vi "TempAlgoTest (SubVI).vi"(0 "Temp":refnum<vi>, 1 "Speed Ind":dbl format="%#_13g", 2 "Motor Speed RPM":refnum<vi>, 3 "Round":T1(ring), 4 "Temp Up In":dbl format="%#_13g", 5 "error in (no error)":errorcluster, 6 "String in":refnum<vi>, 7 "Temp Goal":dbl format="%#_13g", 8 "Stop":refnum<vi>, 9 "Speed Goal":dbl format="%#_13g", 10 "Stop BurnIn":refnum<vi>, 11 "AD Resistor Step":i32=9, 12 "Strin":string, 13 "AccuTemp":dbl=3.0 format="%#_13g") -> (14 "Speed Pass/Fail":bool, 15 "Temp  Pass/Fail":dbl, 16 "Temp Up Out":dbl, 17 "Speed Pass/Fail":dbl, 18 "Temp Pass/Fail":bool, 19 "error out":errorcluster)   [LabVIEW 2017]
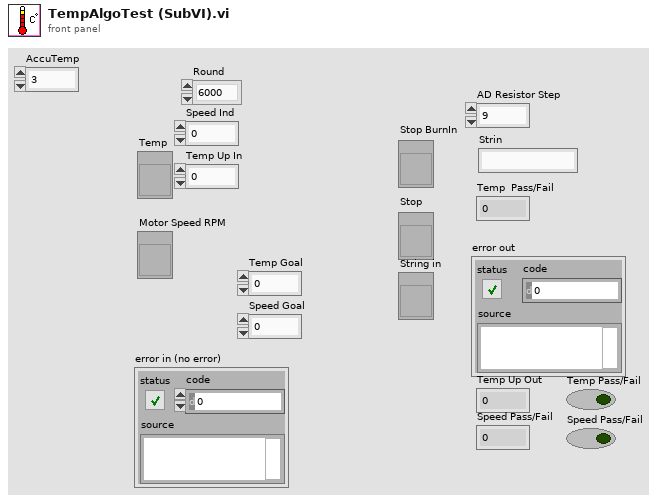
[diagram p1: front panel]
types:
  T1 = enum32{"6000", "11500", "15100", "11500-2", "6000-2"}
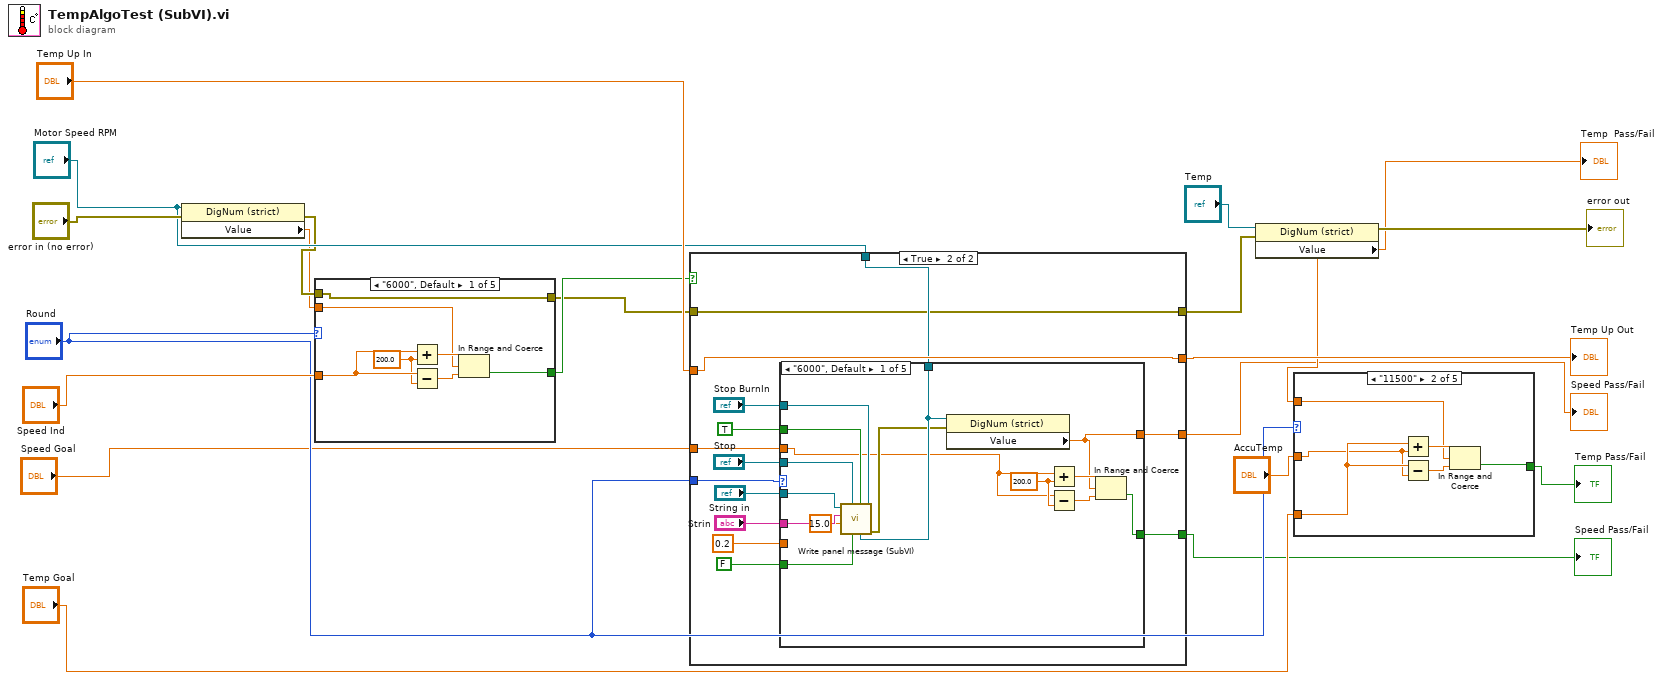
[diagram p0: block diagram]
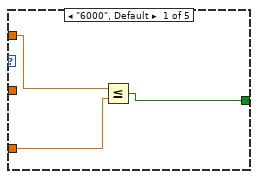
[diagram p2: hidden frame]
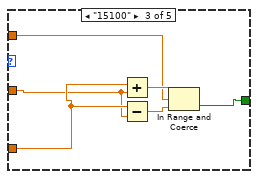
[diagram p3: hidden frame]
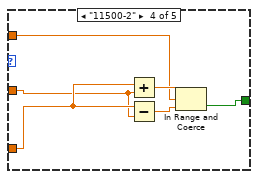
[diagram p4: hidden frame]
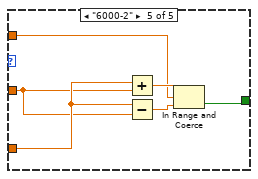
[diagram p5: hidden frame]
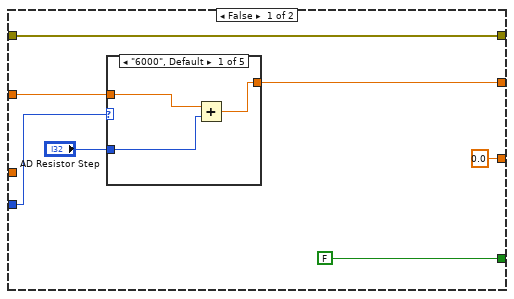
[diagram p6: hidden frame]
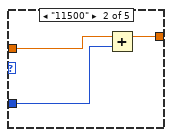
[diagram p7: hidden frame]
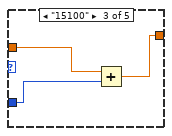
[diagram p8: hidden frame]
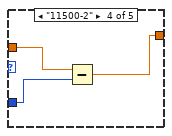
[diagram p9: hidden frame]
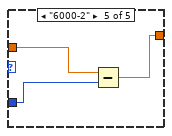
[diagram p10: hidden frame]
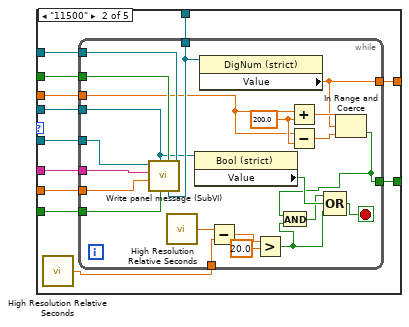
[diagram p11: hidden frame]
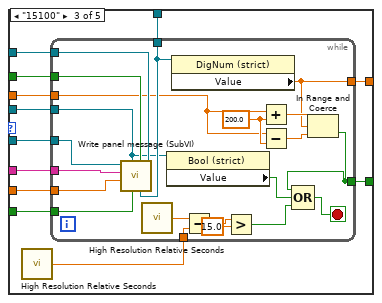
[diagram p12: hidden frame]
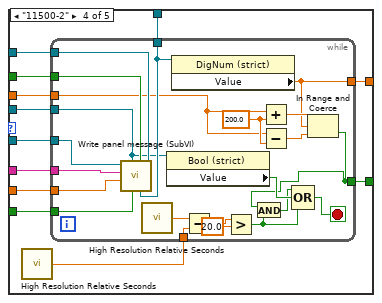
[diagram p13: hidden frame]
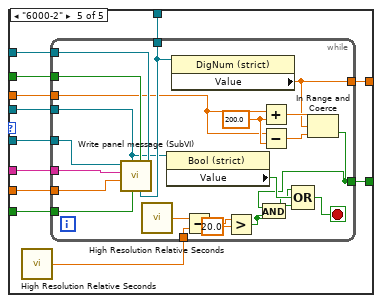
[diagram p14: hidden frame]
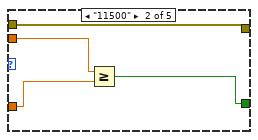
[diagram p15: hidden frame]
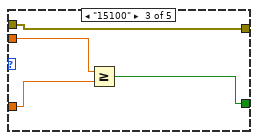
[diagram p16: hidden frame]
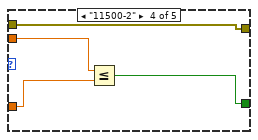
[diagram p17: hidden frame]
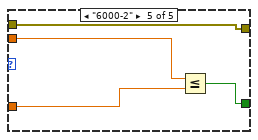
[diagram p18: hidden frame]
diagram:
  n1 = property class="DigNum (strict)"(reference="Motor Speed RPM", error in="error in (no error)") -> (error out=w7:errorcluster, "Value"=w4:dbl)  [unwired: 1 out]
  n2 = case shown="\"6000\", Default" "Round" {
    tunnel: w4 -> [w24 w31 w35 w39 w43]
    tunnel: "Speed Ind" -> [w25 w30 w34 w38 w42]
    tunnel: [w22 w29 w33 w37 w41] -> w15
    tunnel: w7 -> [w21 w28 w32 w36 w40]
    tunnel: [w21 w28 w32 w36 w40] -> w6
    frame "6000", Default {
      w23 = 200.0 ("y")
      n3 = Add(x=w25, y=w23) -> (x+y=w27:dbl)
      n4 = Subtract(x=w25, y=w23) -> (x-y=w26:dbl)
      n5 = In Range and Coerce(upper limit=w27, x=w24, lower limit=w26) -> (In Range?=w22:bool)  [unwired: 1 out]
    }
    frame "11500" {
      n6 = Greater Or Equal?(x=w31, y=w30) -> (x >= y?=w29:bool)
    }
    frame "15100" {
      n7 = Greater Or Equal?(x=w35, y=w34) -> (x >= y?=w33:bool)
    }
    frame "11500-2" {
      n8 = Less Or Equal?(x=w39, y=w38) -> (x <= y?=w37:bool)
    }
    frame "6000-2" {
      n9 = Less Or Equal?(x=w43, y=w42) -> (x <= y?=w41:bool)
    }
  }
  n10 = case shown="True" w15 {
    tunnel: "Temp Up In" -> [w50 w79]
    tunnel: [w49 w79] -> w14
    tunnel: "Motor Speed RPM" -> [_ w71]
    tunnel: "Round" -> [w45 w70]
    tunnel: [FALSE ("rpm 2") w69] -> w8
    tunnel: w6 -> [w47 w68]
    tunnel: [w47 w68] -> w5
    tunnel: "Speed Goal" -> [_ w67]
    tunnel: [0.0 ("Value") w66] -> w2
    frame False {
      n11 = case shown="\"6000\", Default" w45 {
        tunnel: w50 -> [w53 w56 w59 w62 w65]
        tunnel: [w52 w55 w58 w61 w64] -> w49
        tunnel: "AD Resistor Step" -> [w51 w54 w57 w60 w63]
        frame "6000", Default {
          n12 = Add(x=w53, y=w51) -> (x+y=w52:dbl)
        }
        frame "11500" {
          n13 = Add(x=w56, y=w54) -> (x+y=w55:dbl)
        }
        frame "15100" {
          n14 = Add(x=w59, y=w57) -> (x+y=w58:dbl)
        }
        frame "11500-2" {
          n15 = Subtract(x=w62, y=w60) -> (x-y=w61:dbl)
        }
        frame "6000-2" {
          n16 = Subtract(x=w65, y=w63) -> (x-y=w64:dbl)
        }
      }
    }
    frame True {
      n17 = case shown="\"6000\", Default" w70 {
        tunnel: "Stop BurnIn" -> [w92 w106 w140 w173 w207]
        tunnel: TRUE ("rpm 2") -> [w91 w105 w139 w172 w206]
        tunnel: FALSE ("PrintTime") -> [w89 w104 w138 w171 w205]
        tunnel: "Stop" -> [w93 w103 w137 w170 w204]
        tunnel: 0.2 ("Time to wait") -> [_ w102 w136 w169 w203]
        tunnel: "Strin" -> [w90 w101 w135 w168 w202]
        tunnel: "String in" -> [w94 w100 w134 w167 w201]
        tunnel: w71 -> [w88 w99 w133 w166 w200]
        tunnel: [w81 w96 w130 w163 w197] -> w69
        tunnel: w67 -> [w82 w98 w132 w165 w199]
        tunnel: [w80 w97 w131 w164 w198] -> w66
        frame "6000", Default {
          w85 = 200.0 ("y")
          n18 = call "Write panel message (SubVI).vi"("Stop BurnIn"=w92, 4:"rpm"=w88, 5:"rpm"=w91, "PrintTime"=w89, "Stop"=w93, "Time to wait"=15.0, "Strin"=w90, "String in"=w94) -> ("error out"=w87:errorcluster)  [unwired: 3 in]
          n19 = property class="DigNum (strict)"(reference=w88, error in=w87) -> ("Value"=w80:dbl)  [unwired: 2 out]
          n20 = Add(x=w82, y=w85) -> (x+y=w83:dbl)
          n21 = Subtract(x=w82, y=w85) -> (x-y=w84:dbl)
          n22 = In Range and Coerce(upper limit=w83, x=w80, lower limit=w84) -> (In Range?=w81:bool)  [unwired: 1 out]
        }
        frame "11500" {
          n23 = call <vilib>:"High Resolution Relative Seconds.vi"() -> ("relative seconds"=w95:dbl)
          n24 = while {
            tunnel: w106 -> [w128]
            tunnel: w105 -> [w127]
            tunnel: w104 -> [w126]
            tunnel: w103 -> [w121]
            tunnel: w102 -> [w125]
            tunnel: w101 -> [w124]
            tunnel: w100 -> [w123]
            tunnel: w99 -> [w122]
            tunnel: w98 -> [w117]
            tunnel: [w116] -> w97
            tunnel: [w107] -> w96
            tunnel: w95 -> [w112]
            stop <- w115 stop-if-true
            w120 = 200.0 ("y")
            n25 = call "Write panel message (SubVI).vi"("Stop BurnIn"=w128, 4:"rpm"=w122, 5:"rpm"=w127, "PrintTime"=w126, "Stop"=w121, "Time to wait"=w125, "Strin"=w124, "String in"=w123) -> ()  [unwired: 3 in, 1 out]
            n26 = call <vilib>:"High Resolution Relative Seconds.vi"() -> ("relative seconds"=w113:dbl)
            n27 = property class="Bool (strict)"(reference=w121) -> ("Value"=w114:bool)  [unwired: 1 in, 2 out]
            n28 = property class="DigNum (strict)"(reference=w122) -> ("Value"=w116:dbl)  [unwired: 1 in, 2 out]
            n29 = Subtract(x=w113, y=w112) -> (x-y=w111:dbl)
            n30 = Greater?(x=w111, y=20.0) -> (0:w109:bool)
            n31 = Add(x=w117, y=w120) -> (x+y=w118:dbl)
            n32 = Subtract(x=w117, y=w120) -> (x-y=w119:dbl)
            n33 = In Range and Coerce(upper limit=w118, x=w116, lower limit=w119) -> (In Range?=w107:bool)  [unwired: 1 out]
            n34 = And(x=w107, y=w109) -> (x .and. y?=w108:bool)
            n35 = Compound Arithmetic op=OR(w108, w114, w109) -> (w115:bool)
          }
        }
        frame "15100" {
          n36 = call <vilib>:"High Resolution Relative Seconds.vi"() -> ("relative seconds"=w129:dbl)
          n37 = while {
            tunnel: w140 -> [w161]
            tunnel: w139 -> [w160]
            tunnel: w138 -> [w159]
            tunnel: w137 -> [w154]
            tunnel: w136 -> [w158]
            tunnel: w135 -> [w157]
            tunnel: w134 -> [w156]
            tunnel: w133 -> [w155]
            tunnel: w132 -> [w150]
            tunnel: [w149] -> w131
            tunnel: [w147] -> w130
            tunnel: w129 -> [w144]
            stop <- w148 stop-if-true
            w153 = 200.0 ("y")
            n38 = call "Write panel message (SubVI).vi"("Stop BurnIn"=w161, 4:"rpm"=w155, 5:"rpm"=w160, "PrintTime"=w159, "Stop"=w154, "Time to wait"=w158, "Strin"=w157, "String in"=w156) -> ()  [unwired: 3 in, 1 out]
            n39 = call <vilib>:"High Resolution Relative Seconds.vi"() -> ("relative seconds"=w145:dbl)
            n40 = property class="Bool (strict)"(reference=w154) -> ("Value"=w146:bool)  [unwired: 1 in, 2 out]
            n41 = property class="DigNum (strict)"(reference=w155) -> ("Value"=w149:dbl)  [unwired: 1 in, 2 out]
            n42 = Subtract(x=w145, y=w144) -> (x-y=w143:dbl)
            n43 = Greater?(x=w143, y=15.0) -> (0:w141:bool)
            n44 = Add(x=w150, y=w153) -> (x+y=w151:dbl)
            n45 = Subtract(x=w150, y=w153) -> (x-y=w152:dbl)
            n46 = In Range and Coerce(upper limit=w151, x=w149, lower limit=w152) -> (In Range?=w147:bool)  [unwired: 1 out]
            n47 = Compound Arithmetic op=OR(w147, w146, w141) -> (w148:bool)
          }
        }
        frame "11500-2" {
          n48 = call <vilib>:"High Resolution Relative Seconds.vi"() -> ("relative seconds"=w162:dbl)
          n49 = while {
            tunnel: w173 -> [w195]
            tunnel: w172 -> [w194]
            tunnel: w171 -> [w193]
            tunnel: w170 -> [w188]
            tunnel: w169 -> [w192]
            tunnel: w168 -> [w191]
            tunnel: w167 -> [w190]
            tunnel: w166 -> [w189]
            tunnel: w165 -> [w184]
            tunnel: [w183] -> w164
            tunnel: [w174] -> w163
            tunnel: w162 -> [w179]
            stop <- w182 stop-if-true
            w187 = 200.0 ("y")
            n50 = call "Write panel message (SubVI).vi"("Stop BurnIn"=w195, 4:"rpm"=w189, 5:"rpm"=w194, "PrintTime"=w193, "Stop"=w188, "Time to wait"=w192, "Strin"=w191, "String in"=w190) -> ()  [unwired: 3 in, 1 out]
            n51 = call <vilib>:"High Resolution Relative Seconds.vi"() -> ("relative seconds"=w180:dbl)
            n52 = property class="Bool (strict)"(reference=w188) -> ("Value"=w181:bool)  [unwired: 1 in, 2 out]
            n53 = property class="DigNum (strict)"(reference=w189) -> ("Value"=w183:dbl)  [unwired: 1 in, 2 out]
            n54 = Subtract(x=w180, y=w179) -> (x-y=w178:dbl)
            n55 = Greater?(x=w178, y=20.0) -> (0:w175:bool)
            n56 = Add(x=w184, y=w187) -> (x+y=w185:dbl)
            n57 = Subtract(x=w184, y=w187) -> (x-y=w186:dbl)
            n58 = In Range and Coerce(upper limit=w185, x=w183, lower limit=w186) -> (In Range?=w174:bool)  [unwired: 1 out]
            n59 = And(x=w174, y=w175) -> (x .and. y?=w176:bool)
            n60 = Compound Arithmetic op=OR(w176, w181, w175) -> (w182:bool)
          }
        }
        frame "6000-2" {
          n61 = call <vilib>:"High Resolution Relative Seconds.vi"() -> ("relative seconds"=w196:dbl)
          n62 = while {
            tunnel: w207 -> [w229]
            tunnel: w206 -> [w228]
            tunnel: w205 -> [w227]
            tunnel: w204 -> [w222]
            tunnel: w203 -> [w226]
            tunnel: w202 -> [w225]
            tunnel: w201 -> [w224]
            tunnel: w200 -> [w223]
            tunnel: w199 -> [w218]
            tunnel: [w217] -> w198
            tunnel: [w210] -> w197
            tunnel: w196 -> [w213]
            stop <- w216 stop-if-true
            w221 = 200.0 ("y")
            n63 = call "Write panel message (SubVI).vi"("Stop BurnIn"=w229, 4:"rpm"=w223, 5:"rpm"=w228, "PrintTime"=w227, "Stop"=w222, "Time to wait"=w226, "Strin"=w225, "String in"=w224) -> ()  [unwired: 3 in, 1 out]
            n64 = call <vilib>:"High Resolution Relative Seconds.vi"() -> ("relative seconds"=w214:dbl)
            n65 = property class="Bool (strict)"(reference=w222) -> ("Value"=w215:bool)  [unwired: 1 in, 2 out]
            n66 = property class="DigNum (strict)"(reference=w223) -> ("Value"=w217:dbl)  [unwired: 1 in, 2 out]
            n67 = Subtract(x=w214, y=w213) -> (x-y=w212:dbl)
            n68 = Greater?(x=w212, y=20.0) -> (0:w208:bool)
            n69 = Add(x=w218, y=w221) -> (x+y=w219:dbl)
            n70 = Subtract(x=w218, y=w221) -> (x-y=w220:dbl)
            n71 = In Range and Coerce(upper limit=w219, x=w217, lower limit=w220) -> (In Range?=w210:bool)  [unwired: 1 out]
            n72 = And(x=w210, y=w208) -> (x .and. y?=w209:bool)
            n73 = Compound Arithmetic op=OR(w209, w215, w208) -> (w216:bool)
          }
        }
      }
    }
  }
  "Temp Up Out" <- w14
  "Speed Pass/Fail" <- w8
  "Speed Pass/Fail" <- w2
  n74 = property class="DigNum (strict)"(reference="Temp", error in=w5) -> (error out=→"error out":errorcluster, "Value"=w13:dbl)  [unwired: 1 out]
  "Temp  Pass/Fail" <- w13
  n75 = case shown="\"11500\"" "Round" {
    tunnel: w13 -> [w231 w236 w242 w248 w254]
    tunnel: [w232 w234 w240 w246 w252] -> w11
    tunnel: "Temp Goal" -> [w230 w235 w241 w247 w253]
    tunnel: "AccuTemp" -> [_ w233 w239 w245 w251]
    frame "6000", Default {
      n76 = Less Or Equal?(x=w231, y=w230) -> (x <= y?=w232:bool)
    }
    frame "11500" {
      n77 = Add(x=w235, y=w233) -> (x+y=w238:dbl)
      n78 = Subtract(x=w235, y=w233) -> (x-y=w237:dbl)
      n79 = In Range and Coerce(upper limit=w238, x=w236, lower limit=w237) -> (In Range?=w234:bool)  [unwired: 1 out]
    }
    frame "15100" {
      n80 = Add(x=w241, y=w239) -> (x+y=w244:dbl)
      n81 = Subtract(x=w241, y=w239) -> (x-y=w243:dbl)
      n82 = In Range and Coerce(upper limit=w244, x=w242, lower limit=w243) -> (In Range?=w240:bool)  [unwired: 1 out]
    }
    frame "11500-2" {
      n83 = Add(x=w247, y=w245) -> (x+y=w250:dbl)
      n84 = Subtract(x=w247, y=w245) -> (x-y=w249:dbl)
      n85 = In Range and Coerce(upper limit=w250, x=w248, lower limit=w249) -> (In Range?=w246:bool)  [unwired: 1 out]
    }
    frame "6000-2" {
      n86 = Add(x=w253, y=w251) -> (x+y=w256:dbl)
      n87 = Subtract(x=w253, y=w251) -> (x-y=w255:dbl)
      n88 = In Range and Coerce(upper limit=w256, x=w254, lower limit=w255) -> (In Range?=w252:bool)  [unwired: 1 out]
    }
  }
  "Temp Pass/Fail" <- w11
